vi "Create Group from Config.vi"(7 "Group Type (Abstract)":refnum<class "GroupAbstract.lvclass">, 8 "error in (no error)":errorcluster, 10 "Group Config":refnum<class "Group.lvclass">, 11 "Module in":refnum<class "Module.lvclass">) -> (0 "error out":errorcluster, 2 "Group":refnum<class "GroupAbstract.lvclass">, 3 "Module out":refnum<class "Module.lvclass">)   [LabVIEW 2020, in "Volatus.lvlib" / "Module.lvclass"]
uses:
  Module.lvclass
  VolatusConfig/Group/Group.lvclass
  C:/dev/lv20CE/relink/lv-volatus/VolatusConfig/VolatusConfigElement/VolatusConfigElement.lvclass
  lv-vecto/Vecto/GroupAbstract/GroupAbstract.lvclass
  VolatusConfig/VolatusConfigElement/VolatusConfigElement.lvclass/VolatusConfigElement.ctl
  lv-vecto/Vecto/Group/Group.lvclass
  C:/dev/lv20CE/relink/lv-vecto/Vecto/GroupAbstract/GroupAbstract.lvclass
  lv-vecto/Vecto/StringGroup/StringGroup.lvclass
  VolatusConfig/VolatusConfigElement/Element.vi
  VolatusConfig/VolatusConfigElement/Lookup Child by Name.vi
  VolatusConfig/Channel/Channel.lvclass
  lv-cdm/CDM-Config/Config Element/Lookup Child by Name.vi
  lv-cdm/CDM-Config/Config Element/Value (String).vi
  Module.lvclass/Module.ctl
  VolatusConfig/VolatusConfigElement/VolatusConfigElement.lvclass
  C:/dev/lv20CE/relink/lv-volatus/VolatusConfig/Channel/Channel.lvclass
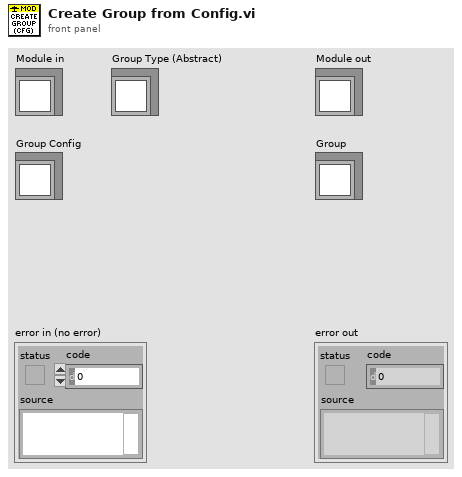
[diagram p1: front panel]
types:
  T1 = typedef "VolatusConfig.lvlib/Group Type.ctl" = enum16{"Double", "String"}
  T2 = typedef "VolatusConfig.lvlib/Endpoint.ctl" = cluster{"Address":string, "Port":u16}
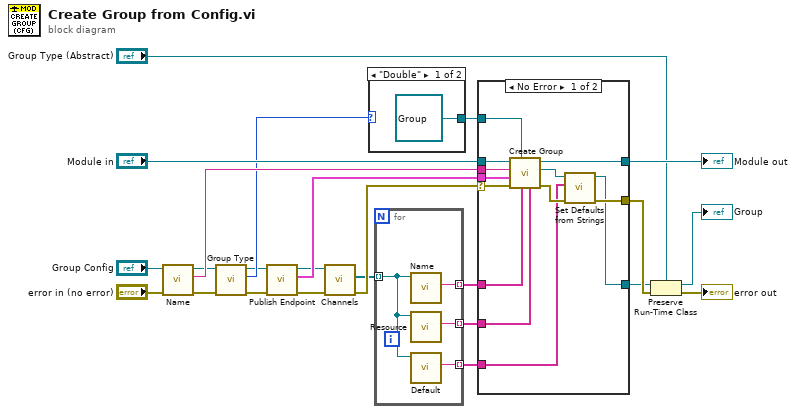
[diagram p0: block diagram]
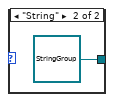
[diagram p2: hidden frame]
diagram:
  n1 = call "Name.vi"("error in (no error)"="error in (no error)", "VolatusConfigElement in"="Group Config") -> ("error out"=w10:errorcluster, "Name"=w18:string, "VolatusConfigElement out"=w17:refnum<class "Group.lvclass">)  [unwired: 7 in]
  n2 = call "Group Type.vi"("error in (no error)"=w10, "Group in"=w17) -> ("error out"=w9:errorcluster, "Group Type"=w16:T1, "Group out"=w14:refnum<class "Group.lvclass">)  [unwired: 7 in]
  n3 = call "Publish Endpoint.vi"("error in (no error)"=w9, "Group in"=w14) -> ("error out"=w8:errorcluster, "Publish Endpoint"=w13:T2, "Group out"=w12:refnum<class "Group.lvclass">)  [unwired: 7 in]
  n4 = call "Channels.vi"("error in (no error)"=w8, "Group in"=w12) -> ("error out"=w22:errorcluster, "Channels"=w7:refnum<class "Channel.lvclass">[])  [unwired: 7 in, 1 out]
  n5 = case shown="\"Double\"" w16 {
    tunnel: [refnum<class "Group.lvclass"> refnum ("Vecto.lvlib:Group.lvclass") refnum<class "StringGroup.lvclass"> refnum ("Vecto.lvlib:StringGroup.lvclass")] -> w15
    frame "Double" {
    }
    frame "String" {
    }
  }
  n6 = for {
    tunnel: w7 -> [w27] mode=indexing
    tunnel: [w30] -> w6 mode=indexing
    tunnel: [w29] -> w5 mode=indexing
    tunnel: [w28] -> w1 mode=indexing
    n7 = call "Name.vi"("VolatusConfigElement in"=w27) -> ("Name"=w29:string)  [unwired: 8 in, 2 out]
    n8 = call "Resource.vi"("Channel in"=w27) -> ("Resource"=w30:string)  [unwired: 8 in, 2 out]
    n9 = call "Default.vi"("Channel in"=w27) -> ("Default"=w28:string)  [unwired: 8 in, 2 out]
  }
  n10 = case shown="No Error" w22 {
    selector: w22 -> [w42 w44]
    tunnel: [w32 w44] -> w24
    tunnel: "Module in" -> [w41 w45]
    tunnel: [w40 w45] -> w20
    tunnel: w18 -> [w39 _]
    tunnel: w15 -> [w38 _]
    tunnel: w13 -> [w37 _]
    tunnel: w6 -> [w36 _]
    tunnel: w5 -> [w35 _]
    tunnel: [w31 _] -> w4
    tunnel: w1 -> [w33 _]
    frame No Error {
      n11 = call "Create Group.vi"("Channel Resources (Unset)"=w36, "Channel Names"=w35, "Group Type"=w38, "error in (no error)"=w42, "Publish Config (Local Only)"=w37, "Group Name"=w39, "Module in"=w41) -> ("error out"=w43:errorcluster, "Group"=w34:refnum<class "GroupAbstract.lvclass">, "Module out"=w40:refnum<class "Module.lvclass">)  [unwired: 2 in]
      n12 = call-dynamic "Set Defaults from Strings.vi"("error in (no error)"=w43, "Default Strings"=w33, "GroupAbstract in"=w34) -> ("error out"=w32:errorcluster, "GroupAbstract out"=w31:refnum<class "GroupAbstract.lvclass">)  [unwired: 7 in]
    }
    frame Error {
    }
  }
  "Module out" <- w20
  n13 = Preserve Run-Time Class(object in=w4, error in=w24, 2:"Group Type (Abstract)") -> (object out=→"Group":refnum<class "GroupAbstract.lvclass">, error out=→"error out":errorcluster)
